vi "CalcSAOXY.vi"(0 "Vx-max":dbl, 1 "Vx-min":dbl, 3 "AOrate":dbl, 6 "xPixels":dbl, 7 "yPixels":dbl) -> (18 "numPixels":dbl, 19 "P":dbl)   [LabVIEW 2015]
panel:
  out "flyback time (us)":dbl
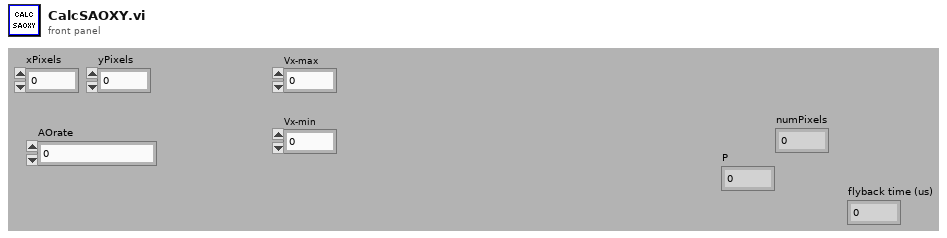
[diagram p1: front panel]
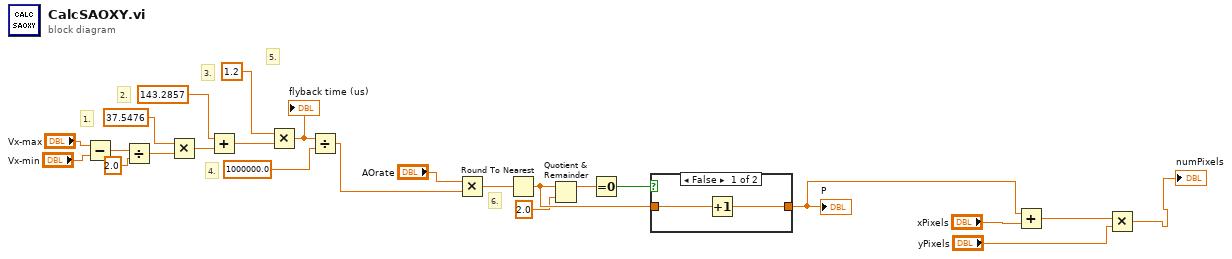
[diagram p0: block diagram]
diagram:
  # "6."
  # "5."
  # "4."
  # "3."
  # "2."
  # "1."
  n1 = Subtract(x="Vx-max", y="Vx-min") -> (x-y=w23:dbl)
  n2 = Divide(x=w23, y=2.0 ("x-y")) -> (x/y=w24:dbl)
  n3 = Multiply(x=37.5476, y=w24) -> (x*y=w8:dbl)
  n4 = Add(x=143.2857, y=w8) -> (x+y=w10:dbl)
  n5 = Multiply(x=1.2, y=w10) -> (x*y=w12:dbl)
  "flyback time (us)" <- w12
  n6 = Divide(x=w12, y=1000000.0 ("x")) -> (x/y=w14:dbl)
  n7 = Multiply(x="AOrate", y=w14) -> (x*y=w15:dbl)
  n8 = Round To Nearest(number=w15) -> (nearest integer value=w19:dbl)
  n9 = Quotient & Remainder(x=w19, y=2.0) -> (x-y*floor(x/y)=w18:dbl)  [unwired: 1 out]
  n10 = Equal To 0?(x=w18) -> (x = 0?=w17:bool)
  n11 = case shown="False" w17 {
    tunnel: [w25 w27] -> w1
    tunnel: w19 -> [w26 w27]
    frame False {
      n12 = Increment(x=w26) -> (x+1=w25:dbl)
    }
    frame True {
    }
  }
  "P" <- w1
  n13 = Add(x=w1, y="xPixels") -> (x+y=w5:dbl)
  n14 = Multiply(x=w5, y="yPixels") -> (x*y=→"numPixels":dbl)
